vi "CRYUnits setup.vi"(0 "unit prefix":string, 1 "Scale visible?":bool=TRUE, 2 "dB/Lin":u16(slide), 5 "Unit:":string="Pa" caption="aa", 7 "dB ref:":dbl=20.0 caption="aa" min=0.0 step=1.0 format="%#.6p", 9 "Custom unit settings":T1={"Custom units dialog?"=TRUE, "Use custom unit?"=TRUE}, 12 "OK":bool, 13 "Common dB ref.":u16(ring)=1 items=["dB", "dBSPL", "dBPa", "dBV", "dBm", "dBu", "dBFS"]) -> (3 "New Scale":u16(ring) items=["Log", "Lin"], 4 "New unit prefix Lin":string="µ", 6 "New unit Lin":string="Pa", 8 "New dB ref":dbl=20.0 format="%.2f", 10 "Common dB #":u16, 11 "Use custom unit out":bool, 14 "Cancelled?":bool, 15 "Common dB":string)   [LabVIEW 2013]
panel:
  in  "Orig Common dB ref":u16=20
  in  "Orig dB ref":dbl=20.0
  in  "Orig Scale":u16(ring) items=["Log", "Lin"]
  in  "Orig unit Lin":string="Pa"
  in  "use custom":bool caption="aa"
  in  "unit prefix:":u16(ring) items=["E", "P", "T", "G", "M", "k", "h", "da", "", "d", "c", "m", "µ", "n", "p", "f", "a"]
  out "Scale":bool caption="aa"
  in  "Cancel":bool
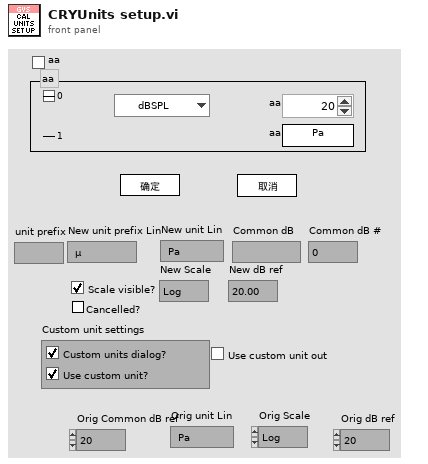
[diagram p1: front panel]
types:
  T1 = cluster{"Custom units dialog?":bool, "Use custom unit?":bool}
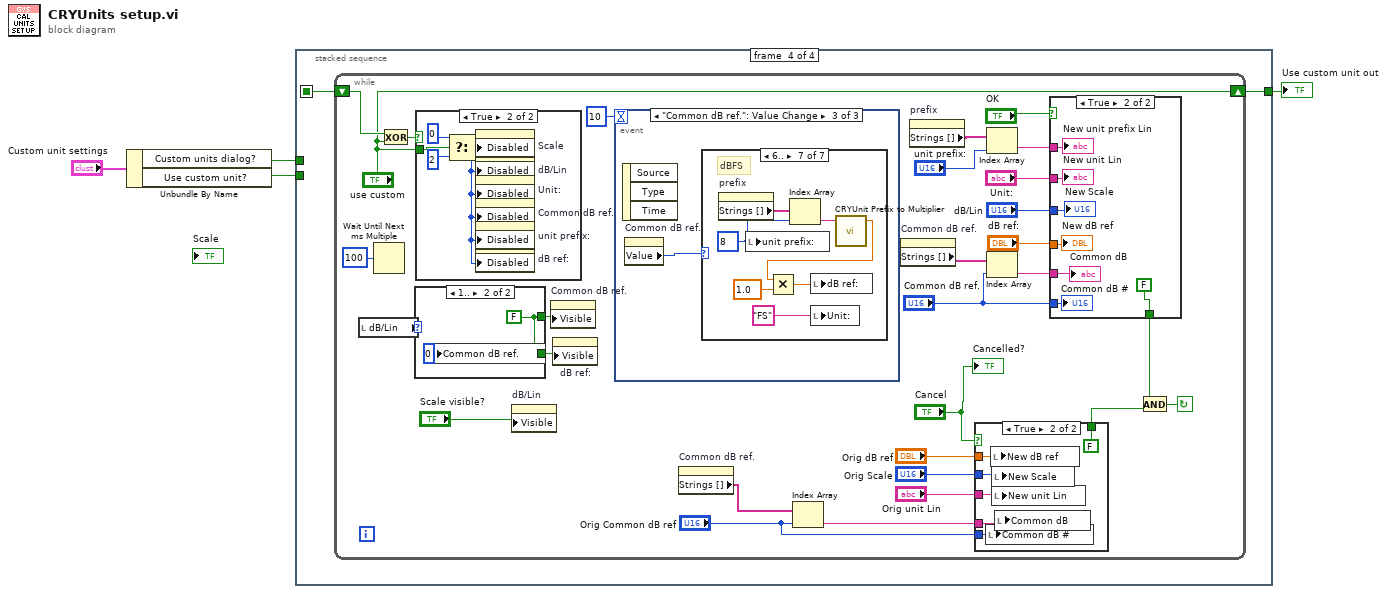
[diagram p0: block diagram]
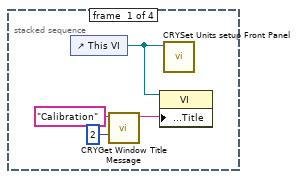
[diagram p2: hidden frame]
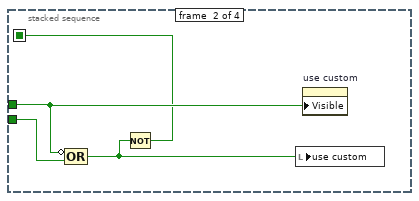
[diagram p3: hidden frame]
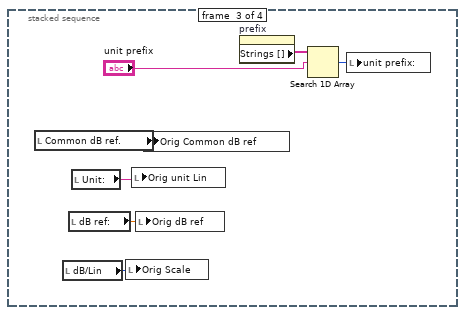
[diagram p4: hidden frame]
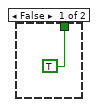
[diagram p5: hidden frame]
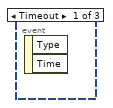
[diagram p6: hidden frame]
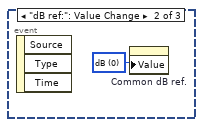
[diagram p7: hidden frame]
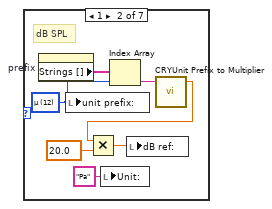
[diagram p9: hidden frame]
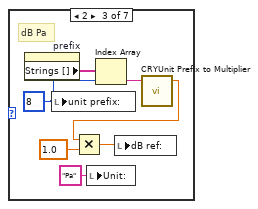
[diagram p10: hidden frame]
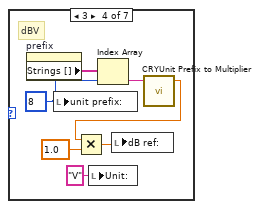
[diagram p11: hidden frame]
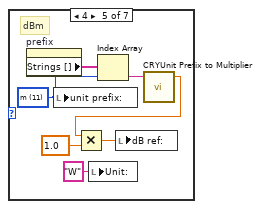
[diagram p12: hidden frame]
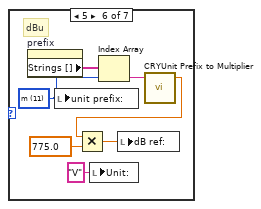
[diagram p13: hidden frame]
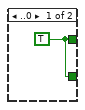
[diagram p15: hidden frame]
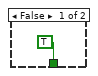
[diagram p16: hidden frame]
diagram:
  n1 = Unbundle By Name("Custom unit settings") -> ("Custom units dialog?"=w3:bool, "Use custom unit?"=w2:bool)
  n2 = stacked-sequence {
    seq-local: [_ w9 _ _] -> [_ _ _ w21]
    tunnel: w3 -> [_ w12 _ _]
    tunnel: w2 -> [_ w11 _ _]
    tunnel: [_ _ _ w20] -> w1
    frame #0 {
      n3 = control-ref of="This VI"() -> (w8:refnum<vi>)
      n4 = call "CRYGet Window Title Message.vi"("No"=2, "Kind"="Calibration") -> ("Multibyte String"=w7:string)  [unwired: 4 in, 5 out]
      n5 = property class="VI"(reference=w8, "Front Panel.Title"=w7) -> ()  [unwired: 1 in, 2 out]
      n6 = call "CRYSet Units setup Front Panel.vi"("Vi Ref"=w8) -> ()  [unwired: 11 in]
    }
    frame #1 {
      n7 = Compound Arithmetic op=OR(invert w12, w11) -> (w10:bool)
      n8 = Not(x=w10) -> (.not. x?=w9:bool)
      n9 = local write "use custom"(w10) -> ()
      n10 = property on="use custom" class="Bool (strict)"("Visible"=w12) -> ()  [unwired: 2 in, 2 out]
    }
    frame #2 {
      n11 = local read "Common dB ref."() -> (w16:u16)
      n12 = local read "dB/Lin"() -> (w13:u16)
      n13 = local read "dB ref:"() -> (w15:dbl)
      n14 = local read "Unit:"() -> (w14:string)
      n15 = local write "Orig Scale"(w13) -> ()
      n16 = local write "Orig unit Lin"(w14) -> ()
      n17 = local write "Orig dB ref"(w15) -> ()
      n18 = local write "Orig Common dB ref"(w16) -> ()
      n19 = property on="prefix" class="Ring (strict)"() -> ("Strings []"=w18:string[])  [unwired: 2 in, 2 out]
      n20 = Search 1D Array(1D array=w18, element="unit prefix") -> (index of element=w17:i32)  [unwired: 1 out]
      n21 = local write "unit prefix:"(w17) -> ()
    }
    frame #3 {
      n22 = while {
        shift-right: ["use custom"] -> w20
        shift-left: w21 -> [w38]
        stop <- w49 continue-if-true
        n23 = local read "dB/Lin"() -> (w45:u16)
        n24 = Wait Until Next ms Multiple(millisecond multiple=100) -> ()  [unwired: 1 out]
        n25 = Exclusive Or(1:"use custom", 2:w38) -> (0:w37:bool)
        n26 = case shown="1.." w45 {
          tunnel: [w106 w108] -> w44
          tunnel: [w106 w108] -> w31
          frame ..0 {
            w106 = TRUE
          }
          frame 1.. {
            w108 = FALSE
            n27 = local write "Common dB ref."(u16 0 ("Common dB ref.")) -> ()
          }
        }
        n28 = case shown="True" w37 {
          tunnel: "use custom" -> [_ w103]
          frame False {
          }
          frame True {
            n29 = Select(t=u8 0 ("Write Attribute"), s=w103, f=u8 2 ("Write Attribute")) -> (s? t:f=w102:u8)
            n30 = property on="Scale" class="Bool (strict)"("Disabled"=w102) -> ()  [unwired: 2 in, 2 out]
            n31 = property on="dB/Lin" class="Slide (strict)"("Disabled"=w102) -> ()  [unwired: 2 in, 2 out]
            n32 = property on="Unit:" class="Str"("Disabled"=w102) -> ()  [unwired: 2 in, 2 out]
            n33 = property on="Common dB ref." class="Ring (strict)"("Disabled"=w102) -> ()  [unwired: 2 in, 2 out]
            n34 = property on="unit prefix:" class="Ring (strict)"("Disabled"=w102) -> ()  [unwired: 2 in, 2 out]
            n35 = property on="dB ref:" class="DigNum (strict)"("Disabled"=w102) -> ()  [unwired: 2 in, 2 out]
          }
        }
        n36 = property on="dB/Lin" class="Slide (strict)"("Visible"="Scale visible?") -> ()  [unwired: 2 in, 2 out]
        n37 = property on="Common dB ref." class="Ring (strict)"("Visible"=w44) -> ()  [unwired: 2 in, 2 out]
        n38 = property on="dB ref:" class="DigNum (strict)"("Visible"=w31) -> ()  [unwired: 2 in, 2 out]
        n39 = event shown="[2] \"Common dB ref.\": Value Change" {
          selector: _ -> [_ _ _]
          dyn-events: _ -> [_ _ _]
          timeout: 10 -> [_ _ _]
          event Timeout {
            n40 = event-data() -> ()  [unwired: 3 out]
          }
          event "dB ref:": Value Change {
            w58 = u16 0 items=["dB", "dBSPL", "dBPa", "dBV", "dBm", "dBu", "dBFS"] ("Common dB ref.")
            n41 = event-data() -> ()  [unwired: 4 out]
            n42 = property on="Common dB ref." class="Ring (strict)"("Value"=w58) -> ()  [unwired: 2 in, 2 out]
          }
          event "Common dB ref.": Value Change {
            n43 = event-data() -> ()  [unwired: 4 out]
            n44 = property on="Common dB ref." class="Ring (strict)"() -> ("Value"=w59:u16)  [unwired: 2 in, 2 out]
            n45 = case shown="6.." w59 {
              frame ..0 {
                # "dB"
              }
              frame 1 {
                w65 = u16 12 items=["E", "P", "T", "G", "M", "k", "h", "da", "", "d", "c", "m", "µ", "n", "p", "f", "a"] ("unit prefix:")
                # "dB SPL"
                n46 = property on="prefix" class="Ring (strict)"() -> ("Strings []"=w66:string[])  [unwired: 2 in, 2 out]
                n47 = local write "unit prefix:"(w65) -> ()
                n48 = local write "Unit:"("Pa" ("unit: Lin")) -> ()
                n49 = Index Array(array=w66, index=w65) -> (element=w64:string)
                n50 = call "CRYUnit Prefix to Multiplier.vi"("unit prefix"=w64) -> ("multiplier"=w62:dbl)  [unwired: 4 out]
                n51 = Multiply(x=w62, y=20.0 ("dB ref:")) -> (x*y=w60:dbl)
                n52 = local write "dB ref:"(w60) -> ()
              }
              frame 2 {
                w71 = u16 8 items=["E", "P", "T", "G", "M", "k", "h", "da", "", "d", "c", "m", "µ", "n", "p", "f", "a"] ("unit prefix:")
                # "dB Pa"
                n53 = property on="prefix" class="Ring (strict)"() -> ("Strings []"=w72:string[])  [unwired: 2 in, 2 out]
                n54 = local write "unit prefix:"(w71) -> ()
                n55 = local write "Unit:"("Pa" ("unit: Lin")) -> ()
                n56 = Index Array(array=w72, index=w71) -> (element=w70:string)
                n57 = call "CRYUnit Prefix to Multiplier.vi"("unit prefix"=w70) -> ("multiplier"=w73:dbl)  [unwired: 4 out]
                n58 = Multiply(x=w73, y=1.0 ("dB ref:")) -> (x*y=w67:dbl)
                n59 = local write "dB ref:"(w67) -> ()
              }
              frame 3 {
                w78 = u16 8 items=["E", "P", "T", "G", "M", "k", "h", "da", "", "d", "c", "m", "µ", "n", "p", "f", "a"] ("unit prefix:")
                # "dBV"
                n60 = property on="prefix" class="Ring (strict)"() -> ("Strings []"=w79:string[])  [unwired: 2 in, 2 out]
                n61 = local write "unit prefix:"(w78) -> ()
                n62 = local write "Unit:"("V" ("unit: Lin")) -> ()
                n63 = Index Array(array=w79, index=w78) -> (element=w77:string)
                n64 = call "CRYUnit Prefix to Multiplier.vi"("unit prefix"=w77) -> ("multiplier"=w80:dbl)  [unwired: 4 out]
                n65 = Multiply(x=w80, y=1.0 ("dB ref:")) -> (x*y=w74:dbl)
                n66 = local write "dB ref:"(w74) -> ()
              }
              frame 4 {
                w85 = u16 11 items=["E", "P", "T", "G", "M", "k", "h", "da", "", "d", "c", "m", "µ", "n", "p", "f", "a"] ("unit prefix:")
                # "dBm"
                n67 = property on="prefix" class="Ring (strict)"() -> ("Strings []"=w86:string[])  [unwired: 2 in, 2 out]
                n68 = local write "unit prefix:"(w85) -> ()
                n69 = local write "Unit:"("W" ("unit: Lin")) -> ()
                n70 = Index Array(array=w86, index=w85) -> (element=w84:string)
                n71 = call "CRYUnit Prefix to Multiplier.vi"("unit prefix"=w84) -> ("multiplier"=w87:dbl)  [unwired: 4 out]
                n72 = Multiply(x=w87, y=1.0 ("dB ref:")) -> (x*y=w81:dbl)
                n73 = local write "dB ref:"(w81) -> ()
              }
              frame 5 {
                w92 = u16 11 items=["E", "P", "T", "G", "M", "k", "h", "da", "", "d", "c", "m", "µ", "n", "p", "f", "a"] ("unit prefix:")
                # "dBu"
                n74 = property on="prefix" class="Ring (strict)"() -> ("Strings []"=w93:string[])  [unwired: 2 in, 2 out]
                n75 = local write "unit prefix:"(w92) -> ()
                n76 = local write "Unit:"("V" ("unit: Lin")) -> ()
                n77 = Index Array(array=w93, index=w92) -> (element=w91:string)
                n78 = call "CRYUnit Prefix to Multiplier.vi"("unit prefix"=w91) -> ("multiplier"=w94:dbl)  [unwired: 4 out]
                n79 = Multiply(x=w94, y=775.0 ("dB ref:")) -> (x*y=w88:dbl)
                n80 = local write "dB ref:"(w88) -> ()
              }
              frame 6.. {
                w99 = u16 8 items=["E", "P", "T", "G", "M", "k", "h", "da", "", "d", "c", "m", "µ", "n", "p", "f", "a"] ("unit prefix:")
                # "dBFS"
                n81 = property on="prefix" class="Ring (strict)"() -> ("Strings []"=w100:string[])  [unwired: 2 in, 2 out]
                n82 = local write "unit prefix:"(w99) -> ()
                n83 = Index Array(array=w100, index=w99) -> (element=w98:string)
                n84 = local write "Unit:"("FS" ("unit: Lin")) -> ()
                n85 = call "CRYUnit Prefix to Multiplier.vi"("unit prefix"=w98) -> ("multiplier"=w101:dbl)  [unwired: 4 out]
                n86 = Multiply(x=w101, y=1.0 ("dB ref:")) -> (x*y=w95:dbl)
                n87 = local write "dB ref:"(w95) -> ()
              }
            }
          }
        }
        n88 = property on="Common dB ref." class="Ring (strict)"() -> ("Strings []"=w25:string[])  [unwired: 2 in, 2 out]
        n89 = Index Array(array=w25, index="Orig Common dB ref") -> (element=w24:string)
        n90 = property on="Common dB ref." class="Ring (strict)"() -> ("Strings []"=w39:string[])  [unwired: 2 in, 2 out]
        n91 = property on="prefix" class="Ring (strict)"() -> ("Strings []"=w42:string[])  [unwired: 2 in, 2 out]
        n92 = case shown="True" "Cancel" {
          tunnel: "Orig dB ref" -> [_ w57]
          tunnel: "Orig Scale" -> [_ w56]
          tunnel: "Orig unit Lin" -> [_ w55]
          tunnel: w24 -> [_ w54]
          tunnel: "Orig Common dB ref" -> [_ w53]
          tunnel: [TRUE FALSE] -> w22
          frame False {
          }
          frame True {
            n93 = local write "Common dB #"(w53) -> ()
            n94 = local write "New dB ref"(w57) -> ()
            n95 = local write "New Scale"(w56) -> ()
            n96 = local write "New unit Lin"(w55) -> ()
            n97 = local write "Common dB"(w54) -> ()
          }
        }
        n98 = Index Array(array=w42, index="unit prefix:") -> (element=w43:string)
        n99 = Index Array(array=w39, index="Common dB ref.") -> (element=w40:string)
        n100 = case shown="True" "OK" {
          tunnel: "dB ref:" -> [_ w116]
          tunnel: w43 -> [_ w115]
          tunnel: "Unit:" -> [_ w114]
          tunnel: [TRUE FALSE] -> w33
          tunnel: "dB/Lin" -> [_ w112]
          tunnel: w40 -> [_ w111]
          tunnel: "Common dB ref." -> [_ w110]
          frame False {
          }
          frame True {
            "New unit prefix Lin" <- w115
            "New unit Lin" <- w114
            "New dB ref" <- w116
            "New Scale" <- w112
            "Common dB" <- w111
            "Common dB #" <- w110
          }
        }
        n101 = And(x=w33, y=w22) -> (x .and. y?=w49:bool)
        "Cancelled?" <- "Cancel"
      }
    }
  }
  "Use custom unit out" <- w1
